vi "Concatenate Array.vi"(1 "a":refnum<class "Bytestream.lvclass">[](array[class])) -> (0 "c":refnum<class "Bytestream.lvclass">)   [LabVIEW 2020, in "NI_Bytestream.lvlib" / "Bytestream.lvclass"]
uses:
  <vilib>/Array/Bytestream/Bytestream.lvclass
  <vilib>/Array/Bytestream/Datum.ctl
  <vilib>/Array/Bytestream/Bytestream.lvclass/Bytestream.ctl
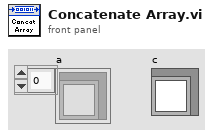
[diagram p1: front panel]
types:
  T1 = typedef "NI_Bytestream.lvlib/Bytestream.lvclass/Datum.ctl" = cluster{"array":u8[], "index":i32}
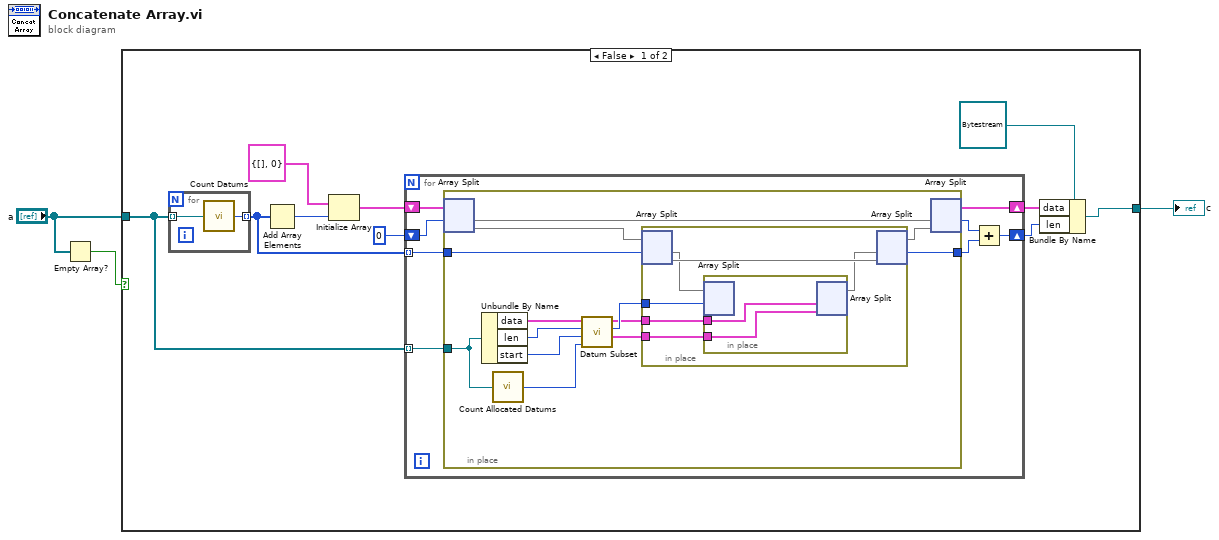
[diagram p0: block diagram]
diagram:
  n1 = Empty Array?(array="a") -> (empty?=w1:bool)
  n2 = case shown="False" w1 {
    tunnel: [w6 _] -> w3
    tunnel: "a" -> [w4 _]
    frame False {
      n3 = for {
        tunnel: w4 -> [w44] mode=indexing
        tunnel: [w43] -> w9 mode=indexing
        n4 = call <vilib>:"Count Datums.vi"("bytestream"=w44) -> ("datums"=w43:i32)
      }
      n5 = Add Array Elements(numeric array=w9) -> (sum=w13:i32)
      n6 = Initialize Array(T1 {"array"=[], "index"=0} ("datum"), w13) -> (w11:T1[])
      n7 = for {
        shift-right: [w14] -> w5
        shift-left: 0 -> [w20]
        tunnel: w9 -> [w19] mode=indexing
        tunnel: w4 -> [w18] mode=indexing
        shift-right: [w15] -> w7
        shift-left: w11 -> [w21]
        n8 = in-place {
          in-place-border: w19 -> [w32]
          in-place-border: w18 -> [w24]
          in-place-border: [w30] -> w16
          n9 = in-place-split #1(w21, w20) -> (w34:T1[], w33:T1[])
          n10 = Unbundle By Name(w24) -> ("data"=w29:T1[], "len"=w23:i32, "start"=w22:i32)
          n11 = call <vilib>:"Count Allocated Datums.vi"("bytestream"=w24) -> ("datums"=w28:i32)
          n12 = call <vilib>:"Datum Subset.vi"("limit size"=w28, "start"=w22, "len"=w23, "data"=w29) -> ("datums out"=w25:T1[], "count of datums 1"=w27:i32, "datums 1"=w26:T1[])  [unwired: 4 in, 1 out]
          n13 = in-place {
            in-place-border: w27 -> [w38]
            in-place-border: w26 -> [w37]
            in-place-border: w25 -> [w36]
            n14 = in-place-split #2(w33, w32) -> (w39:T1[], w40:T1[])
            n15 = in-place {
              in-place-border: w37 -> [w42]
              in-place-border: w36 -> [w41]
              n16 = in-place-split #3(w39, w38) -> ()  [unwired: 2 out]
              n17 = in-place-split #3(w42, w41) -> (w35:T1[])  [unwired: 1 out]
            }
            n18 = in-place-split #2(w35, w40) -> (w31:T1[], w30:i32)
          }
          n19 = in-place-split #1(w34, w31) -> (w15:T1[], w17:i32)
        }
        n20 = Add(x=w17, y=w16) -> (x+y=w14:i32)
      }
      n21 = Bundle By Name(cluster=refnum<class "Bytestream.lvclass"> refnum ("Bytestream.lvclass"), "data"=w7, "len"=w5) -> (w6:refnum<class "Bytestream.lvclass">)
    }
    frame True {
    }
  }
  "c" <- w3
